vi "QSend.vi"(8 "error in (no error)":errorcluster, 10 "Data":variant, 11 "Command":string) -> (0 "error out":errorcluster)   [LabVIEW 2020, in "SensorInterface.lvlib"]
doc: "Sends a message to the owning module"
uses:
  SensorInterface.lvlib
  Controls/QMessage.ctl
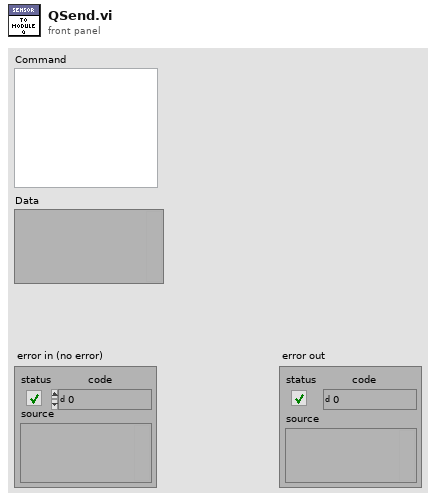
[diagram p1: front panel]
types:
  T1 = typedef "SensorInterface.lvlib/QMessage.ctl" = cluster{"Command":string, "Data":variant}
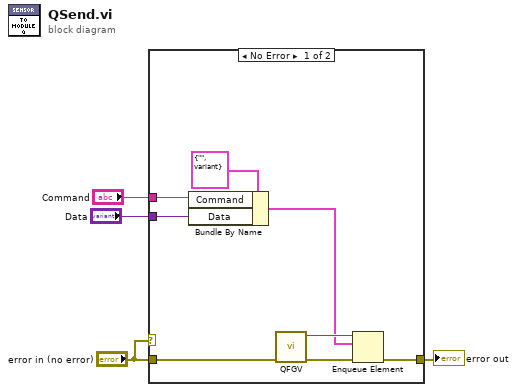
[diagram p0: block diagram]
diagram:
  n1 = case shown="No Error" "error in (no error)" {
    tunnel: [w9 w13] -> w4
    tunnel: "error in (no error)" -> [w5 w13]
    tunnel: "Command" -> [w6 _]
    tunnel: "Data" -> [w7 _]
    frame No Error {
      n2 = Bundle By Name(cluster=T1 {"Command"="", "Data"=variant(errorcluster {"status"=FALSE, "code"=0, "source"=""})}, "Command"=w6, "Data"=w7) -> (w8:T1)
      n3 = call "QFGV.vi"("error in (no error)"=w5) -> ("error out"=w12:errorcluster, "ModuleQ"=w10:refnum<queue>)  [unwired: 9 in]
      n4 = Enqueue Element(queue=w10, element=w8, error in (no error)=w12) -> (error out=w9:errorcluster)  [unwired: 1 in, 2 out]
    }
    frame Error {
    }
  }
  "error out" <- w4
